vi "ProcessState-WaitOnRunning.vi"(2 "PROCESS":string, 9 "error in (no error)":errorcluster) -> (1 "timed out?":bool, 6 "error out":errorcluster)   [LabVIEW 2009]
uses:
  ProcessState.ctl
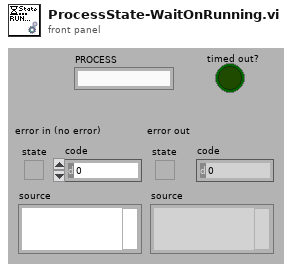
[diagram p1: front panel]
types:
  T1 = typedef "ProcessState.ctl" = enum16{"STARTING", "RUNNING", "STOPPING", "STOPPPED"}
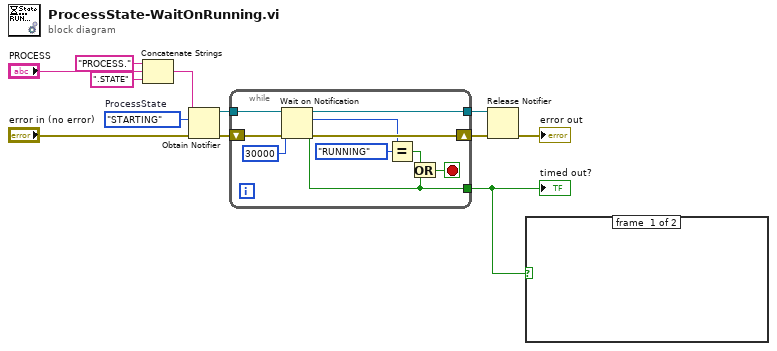
[diagram p0: block diagram]
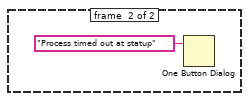
[diagram p2: hidden frame]
diagram:
  w10 = ProcessState."STARTING"  # ProcessState
  n1 = Concatenate Strings("PROCESS." ("chaîne"), "PROCESS", ".STATE" ("chaîne")) -> (w12:string)
  n2 = Obtain Notifier(name (unnamed)=w12, notification data type=w10, error in (no error)="error in (no error)") -> (notifier out=w6:refnum<notifier>, error out=w7:errorcluster)  [unwired: 1 in, 1 out]
  n3 = while {
    tunnel: w6 -> [w21]
    tunnel: [w17] -> w4
    shift-right: [w20] -> w5
    shift-left: w7 -> [w22]
    tunnel: [w13] -> w1
    stop <- w14 stop-if-true
    n4 = Wait on Notification(notifier=w21, timeout in ms (-1)=30000 ("timeout en ms (-1)"), error in (no error)=w22) -> (notifier out=w17:refnum<notifier>, notification=w19:T1, timed out?=w13:bool, error out=w20:errorcluster)  [unwired: 1 in]
    n5 = Equal?(x=w19, y=ProcessState."RUNNING" ("ProcessState")) -> (x = y?=w15:bool)
    n6 = Or(x=w15, y=w13) -> (x .or. y?=w14:bool)
  }
  "timed out?" <- w1
  n7 = Release Notifier(notifier=w4, error in (no error)=w5) -> (error out=→"error out":errorcluster)  [unwired: 1 in, 2 out]
  n8 = case shown="True" w1 {
    frame #0 {
    }
    frame #1 {
      n9 = One Button Dialog(message="Process timed out at statup") -> ()  [unwired: 1 in, 1 out]
    }
  }
